vi "acquisition_test.vi"() -> ()   [LabVIEW 2013, in "main.lvlib"]
uses:
  main.lvlib
  <vilib>/DAQmx/read.llb/DAQmx Read (Analog 1D DBL NChan 1Samp).vi
  <vilib>/Utility/file.llb/Write To Spreadsheet File (DBL).vi
  <vilib>/DAQmx/create/channels.llb/DAQmx Create Channel (AI-Voltage-Basic).vi
  <vilib>/DAQmx/miscellaneous.llb/DAQmx Fill In Error Info.vi
panel:
  out "Tryk":dbl(graph)
  in  "StopBtn":bool
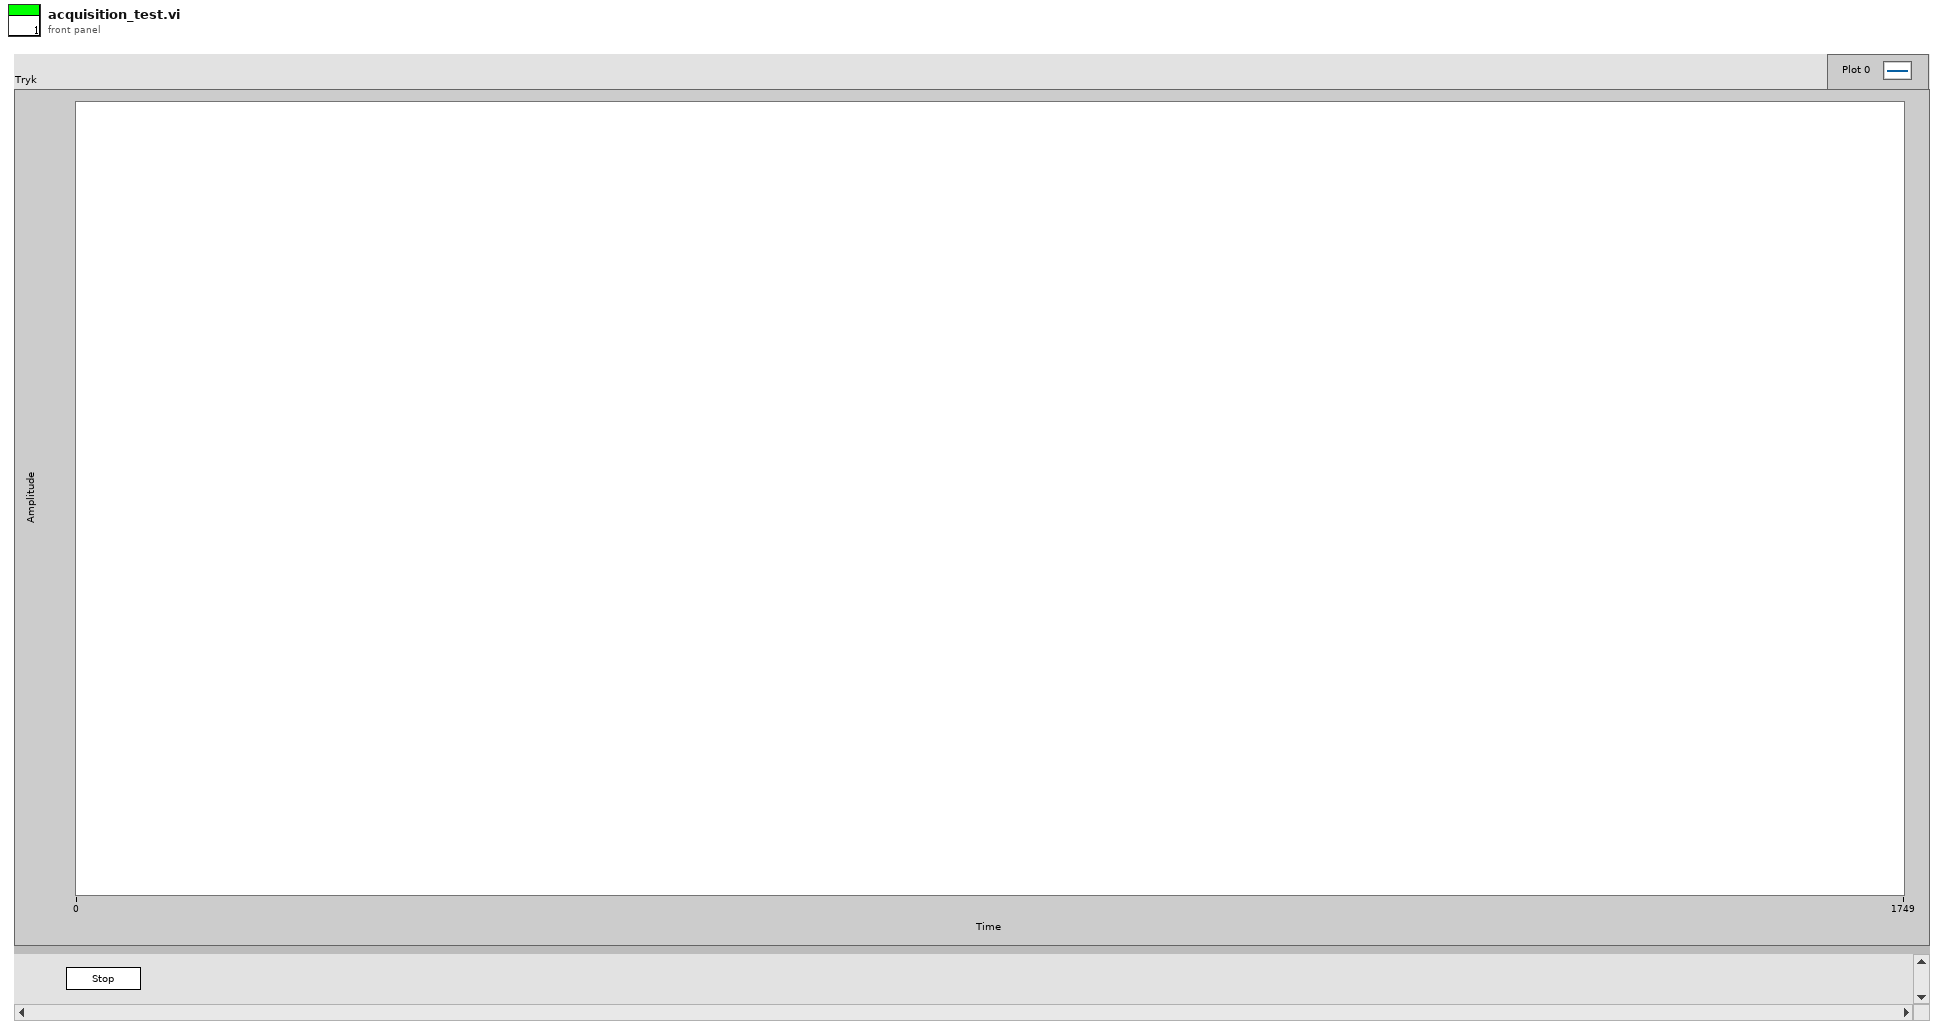
[diagram p1: front panel]
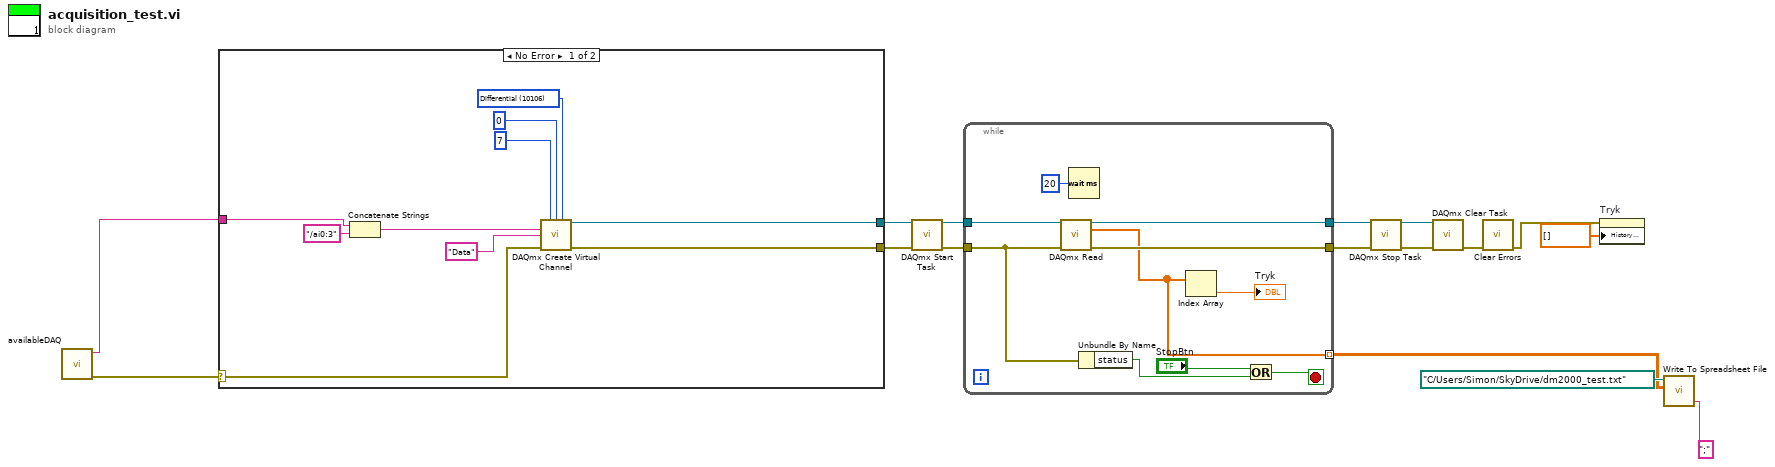
[diagram p0: block diagram]
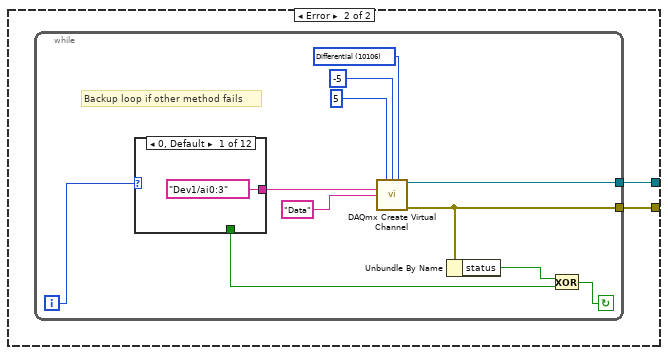
[diagram p2: hidden frame]
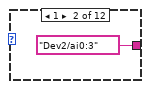
[diagram p3: hidden frame]
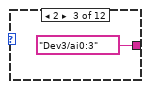
[diagram p4: hidden frame]
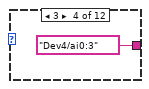
[diagram p5: hidden frame]
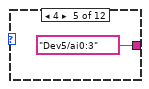
[diagram p6: hidden frame]
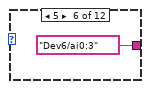
[diagram p7: hidden frame]
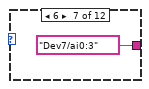
[diagram p8: hidden frame]
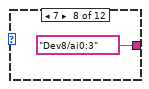
[diagram p9: hidden frame]
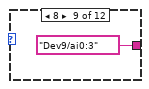
[diagram p10: hidden frame]
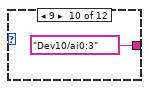
[diagram p11: hidden frame]
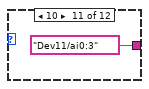
[diagram p12: hidden frame]
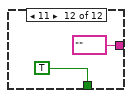
[diagram p13: hidden frame]
diagram:
  n1 = call "availableDAQ.vi"() -> ("error out"=w6:errorcluster, "DAQmx Device Name"=w5:tag)  [unwired: 10 in]
  n2 = case shown="No Error" w6 {
    selector: w6 -> [w21 _]
    tunnel: [w17 w28] -> w4
    tunnel: [w22 w27] -> w3
    tunnel: w5 -> [w18 _]
    frame No Error {
      w23 = 10106 items=["default"=-1, "RSE"=10083, "NRSE"=10078, "Differential"=10106, "Pseudodifferential"=12529] ("input terminal configuration")
      n3 = Concatenate Strings(w18, "/ai0:3" ("string")) -> (w20:string)
      n4 = call-poly <vilib>:"DAQmx Create Virtual Channel.vi"("maximum value"=7, "minimum value"=0, "input terminal configuration"=w23, "physical channels"=w20, "name to assign"="Data", "error in"=w21) -> ("task out"=w17:refnum<k21>, "error out"=w22:errorcluster)  [unwired: 8 in]
    }
    frame Error {
      n5 = while {
        tunnel: [w30] -> w28
        tunnel: [w29] -> w27
        i -> [w34]
        stop <- w33 continue-if-true
        w36 = 10106 items=["default"=-1, "RSE"=10083, "NRSE"=10078, "Differential"=10106, "Pseudodifferential"=12529] ("input terminal configuration")
        # "Backup loop if other method fails"
        n6 = case shown="0, Default" w34 {
          tunnel: [tag "Dev1/ai0:3" ("physical channels") tag "Dev2/ai0:3" ("physical channels") tag "Dev3/ai0:3" ("physical channels") tag "Dev4/ai0:3" ("physical channels") tag "Dev5/ai0:3" ("physical channels") tag "Dev6/ai0:3" ("physical channels") tag "Dev7/ai0:3" ("physical channels") tag "Dev8/ai0:3" ("physical channels") tag "Dev9/ai0:3" ("physical channels") tag "Dev10/ai0:3" ("physical channels") tag "Dev11/ai0:3" ("physical channels") tag "" ("physical channels")] -> w35
          tunnel: [_ _ _ _ _ _ _ _ _ _ _ TRUE] -> w31
          frame 0, Default {
          }
          frame 1 {
          }
          frame 2 {
          }
          frame 3 {
          }
          frame 4 {
          }
          frame 5 {
          }
          frame 6 {
          }
          frame 7 {
          }
          frame 8 {
          }
          frame 9 {
          }
          frame 10 {
          }
          frame 11 {
          }
        }
        n7 = call-poly <vilib>:"DAQmx Create Virtual Channel.vi"("maximum value"=5, "minimum value"=-5, "input terminal configuration"=w36, "physical channels"=w35, "name to assign"="Data") -> ("task out"=w30:refnum<k21>, "error out"=w29:errorcluster)  [unwired: 9 in]
        n8 = Unbundle By Name(w29) -> ("status"=w32:bool)
        n9 = Exclusive Or(1:w31, 2:w32) -> (0:w33:bool)
      }
    }
  }
  n10 = call <vilib>:"DAQmx Start Task.vi"("task/channels in"=w4, "error in"=w3) -> ("task out"=w16:refnum<k21>, "error out"=w15:errorcluster)  [unwired: 12 in]
  n11 = while {
    tunnel: w16 -> [w61]
    tunnel: w15 -> [w56]
    tunnel: [w60] -> w12
    tunnel: [w59] -> w11
    tunnel: [w53] -> w1 mode=indexing
    stop <- w57 stop-if-true
    n12 = call-poly <vilib>:"DAQmx Read.vi"("task/channels in"=w61, "error in"=w56) -> ("task out"=w60:refnum<k21>, "data"=w53:dbl[], "error out"=w59:errorcluster)  [unwired: 11 in]
    n13 = Wait (ms)(milliseconds to wait=u32 20) -> ()  [unwired: 1 out]
    n14 = Unbundle By Name(w56) -> ("status"=w55:bool)
    n15 = Index Array(array=w53) -> (element=→"Tryk":dbl)  [unwired: 1 in]
    n16 = Or(x="StopBtn", y=w55) -> (x .or. y?=w57:bool)
  }
  n17 = call <vilib>:"DAQmx Stop Task.vi"("task/channels in"=w12, "error in"=w11) -> ("task out"=w14:refnum<k21>, "error out"=w13:errorcluster)  [unwired: 12 in]
  n18 = call <vilib>:"DAQmx Clear Task.vi"("task in"=w14, "error in"=w13) -> ("error out"=w10:errorcluster)  [unwired: 13 in]
  n19 = call <vilib>:"Clear Errors.vi"("error in (no error)"=w10) -> ("error out"=w9:errorcluster)  [unwired: 6 in]
  n20 = property on="Tryk" class="WFChart (strict)"(error in=w9, "History Data"=dbl[] []) -> ()  [unwired: 1 in, 2 out]
  n21 = call-poly <vilib>:"Write To Spreadsheet File.vi"("delimiter (\\t)"=";" ("delimiter (\\t)"), "2D data"=w1, "file path (dialog if empty)"=path "C:/Users/Simon/SkyDrive/dm2000_test.txt") -> ()  [unwired: 5 in, 1 out]
